vi "MaskArrayValueGreyscale.vi"(1 "Array In":u8[][](array[numeric])) -> (0 "Array out":u8[][](array[numeric]))   [LabVIEW 2020, in "test.lvlib" / "Image.lvclass"]
uses:
  Image.lvclass
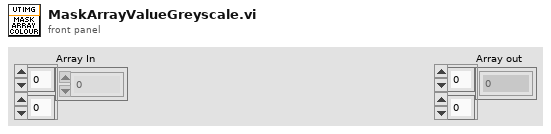
[diagram p1: front panel]
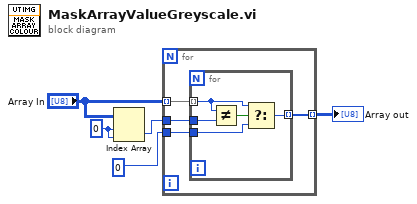
[diagram p0: block diagram]
diagram:
  w3 = 0 ("index (row)")
  n1 = Index Array(array="Array In", index (row)=w3, index (col)=w3) -> (element=w2:u8)
  n2 = for {
    tunnel: "Array In" -> [w9] mode=indexing
    tunnel: w2 -> [w8]
    tunnel: [w7] -> w5 mode=indexing
    tunnel: u8 0 -> [w6]
    n3 = for {
      tunnel: w9 -> [w10] mode=indexing
      tunnel: w8 -> [w13]
      tunnel: [w12] -> w7 mode=indexing
      tunnel: w6 -> [w11]
      n4 = Not Equal?(x=w10, y=w13) -> (x != y?=w14:bool)
      n5 = Select(t=w10, s=w14, f=w11) -> (s? t:f=w12:u8)
    }
  }
  "Array out" <- w5
